vi "Add Database.vi"(7 "Highlight? (F)":bool, 8 "error in":errorcluster, 9 "Path":path, 10 "Name":string, 11 "Database section Ref":T1 format="%.0x") -> (0 "error out":errorcluster, 3 "Database Ref out":T1 format="%.0x")   [LabVIEW 2020, in "Communication Bus Template Scripting.lvlib"]
uses:
  Communication Bus Template Scripting.lvlib
  <vilib>/NI VeriStand/Custom Device API/Custom Device Item Ref.ctl
  System Explorer/Constants.vi
  <vilib>/NI VeriStand/Custom Device API/Set Item Property (Path).vi
  <vilib>/NI VeriStand/Custom Device API/Custom Device API.lvlib
  System Explorer/Implementation.lvlib
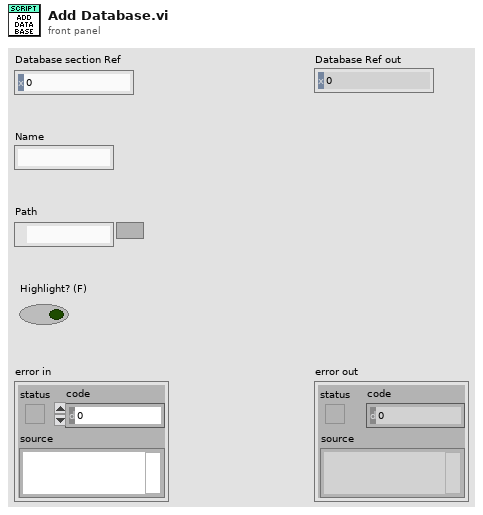
[diagram p1: front panel]
types:
  T1 = typedef "Custom Device API.lvlib/Custom Device Item Ref.ctl" = u64
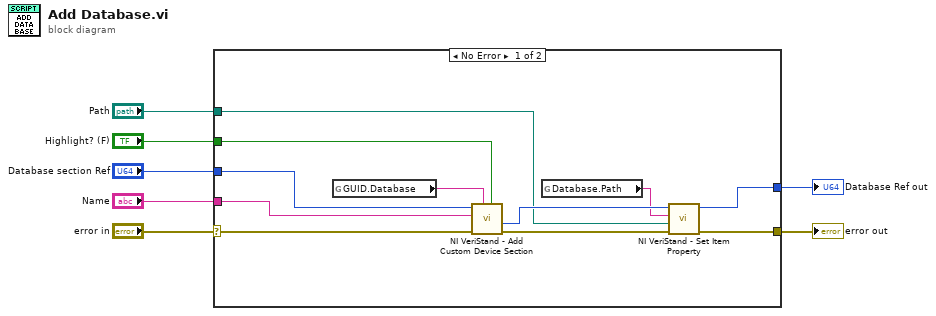
[diagram p0: block diagram]
diagram:
  n1 = case shown="No Error" "error in" {
    selector: "error in" -> [w11 w19]
    tunnel: "Name" -> [w16 _]
    tunnel: "Database section Ref" -> [w15 _]
    tunnel: [w14 w19] -> w5
    tunnel: "Path" -> [w13 _]
    tunnel: "Highlight? (F)" -> [w12 _]
    tunnel: [w10 _] -> w1
    frame No Error {
      n2 = global read "Constants.vi" "GUID.Database"() -> (w9:string)
      n3 = call <vilib>:"NI VeriStand - Add Custom Device Section.vi"("Highlight? (F)"=w12, "GUID (Default Section)"=w9, "error in (no error)"=w11, "Section Name"=w16, "Parent Ref in"=w15) -> ("error out"=w17:errorcluster, "Section Ptr"=w18:T1)  [unwired: 3 in, 2 out]
      n4 = global read "Constants.vi" "Database.Path"() -> (w8:string)
      n5 = call-poly <vilib>:"NI VeriStand - Set Item Property.vi"("error in (no error)"=w17, "Value"=w13, "Property Name"=w8, "Item Ref in"=w18) -> ("error out"=w14:errorcluster, "Item Ref out"=w10:T1)  [unwired: 5 in, 1 out]
    }
    frame Error {
    }
  }
  "error out" <- w5
  "Database Ref out" <- w1
